vi "2-to-4-decoder-labview-vi.vi"() -> ()   [LabVIEW 2012]
panel:
  out "0":bool=TRUE
  out "1":bool=TRUE
  out "2":bool=TRUE
  out "3":bool=TRUE
  in  "INPUT 1":bool=TRUE
  in  "INPUT 0":bool=TRUE
  # "2 - 4 Decoder\nNon-inverted"
  # "Enabled"
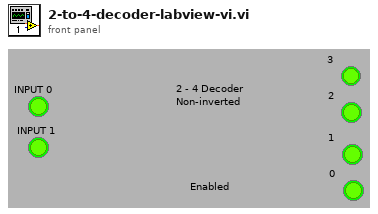
[diagram p1: front panel]
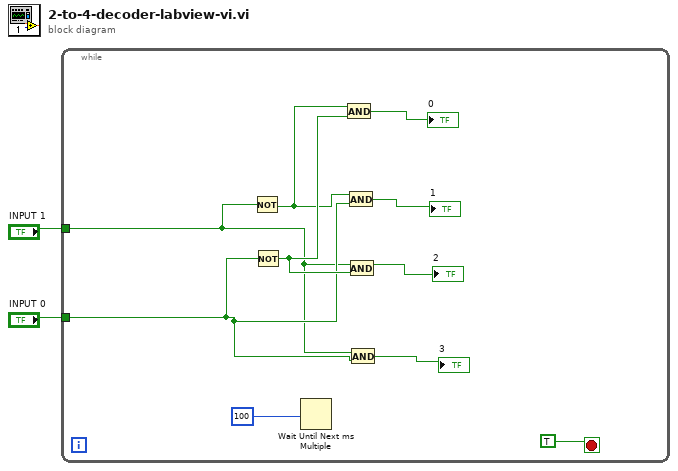
[diagram p0: block diagram]
diagram:
  n1 = while {
    tunnel: "INPUT 0" -> [w4]
    tunnel: "INPUT 1" -> [w3]
    stop <- TRUE stop-if-true
    n2 = Not(x=w3) -> (.not. x?=w11:bool)
    n3 = Not(x=w4) -> (.not. x?=w12:bool)
    n4 = Wait Until Next ms Multiple(millisecond multiple=100) -> ()  [unwired: 1 out]
    n5 = And(x=w11, y=w12) -> (x .and. y?=→"0":bool)
    n6 = And(x=w11, y=w4) -> (x .and. y?=→"1":bool)
    n7 = And(x=w3, y=w12) -> (x .and. y?=→"2":bool)
    n8 = And(x=w3, y=w4) -> (x .and. y?=→"3":bool)
  }
